vi "Initialize.vi"(6 "optional":variant, 8 "error in (no error)":errorcluster, 11 "Tree in":refnum<class "Tree.lvclass">) -> (0 "error out":errorcluster, 3 "Tree out":refnum<class "Tree.lvclass">)   [LabVIEW 2009, in "Tree.lvclass"]
uses:
  Tree.lvclass
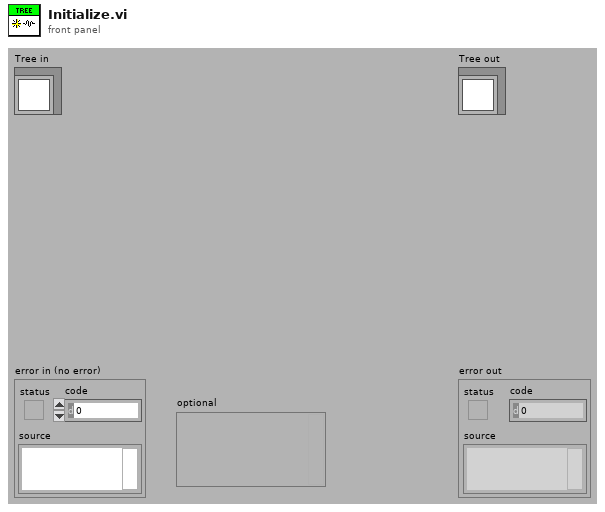
[diagram p1: front panel]
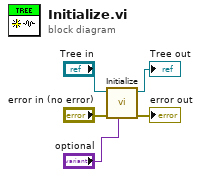
[diagram p0: block diagram]
diagram:
  n1 = call-parent "Initialize.vi"("optional"="optional", "error in (no error)"="error in (no error)", "Structure in"="Tree in") -> ("error out"=→"error out":errorcluster, "Structure out"=→"Tree out":refnum<class "Tree.lvclass">)  [unwired: 7 in]
